vi "Insert Element at Index.vi"(0 "Variant (Cluster) in":variant, 5 "Name":string, 7 "element":variant, 9 "index":i32, 11 "error in (no error)":errorcluster) -> (4 "Variant (Cluster) out":variant, 15 "error out":errorcluster)   [LabVIEW 2017, in "Advanced Variant Tools.lvlib"]
uses:
  Advanced Variant Tools.lvlib
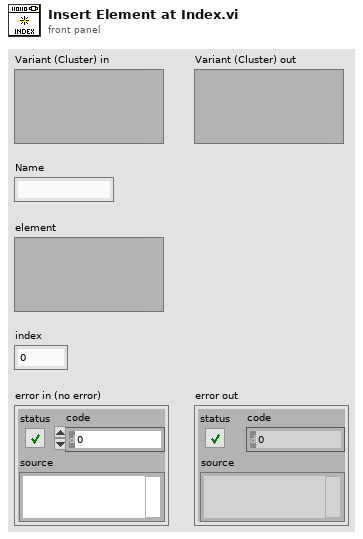
[diagram p1: front panel]
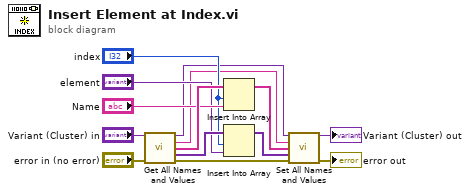
[diagram p0: block diagram]
diagram:
  n1 = call "Get All Names and Values.vi"("Variant (Cluster) In"="Variant (Cluster) in", "error in"="error in (no error)") -> ("Variant (Cluster) Out"=w1:variant, "Name"=w2:string, "Element Names"=w9:string[], "Values"=w6:variant[], "error out"=w13:errorcluster)  [unwired: 9 in]
  n2 = Insert Into Array(array=w9, index="index", new element="Name") -> (w7:string[])
  n3 = Insert Into Array(array=w6, index="index", new element="element") -> (w3:variant[])
  n4 = call "Set All Names and Values.vi"("Variant (Cluster) In"=w1, "Name"=w2, "Element Names"=w7, "values"=w3, "error in"=w13) -> ("Variant (Cluster) Out"=→"Variant (Cluster) out":variant, "error out"=→"error out":errorcluster)  [unwired: 9 in]
